vi "Dir Buttons.vi"(1 "Direction 2":T2) -> (0 "Buttons Control":T1)   [LabVIEW 2015]
uses:
  DIR GAME.ctl
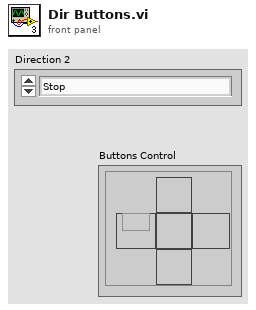
[diagram p1: front panel]
types:
  T1 = cluster{"Front":bool, "Right":bool, "Back":bool, "Left":bool, "Stop":bool}
  T2 = typedef "DIR GAME.ctl" = enum16{"Stop", "Front", "FR", "Right", "BR", "Back", "BL", "Left", "FL"}
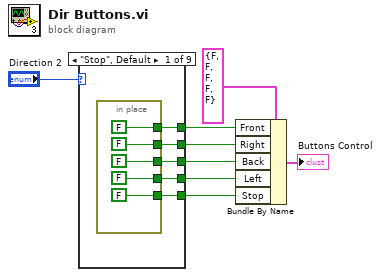
[diagram p0: block diagram]
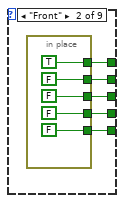
[diagram p2: hidden frame]
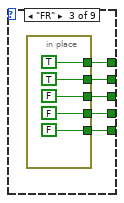
[diagram p3: hidden frame]
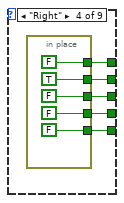
[diagram p4: hidden frame]
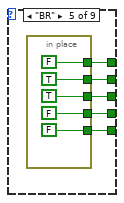
[diagram p5: hidden frame]
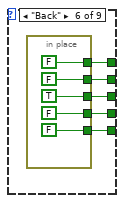
[diagram p6: hidden frame]
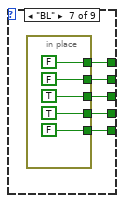
[diagram p7: hidden frame]
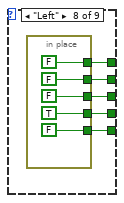
[diagram p8: hidden frame]
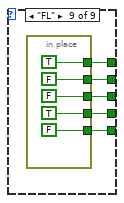
[diagram p9: hidden frame]
diagram:
  n1 = case shown="\"Stop\", Default" "Direction 2" {
    tunnel: [w13 w23 w33 w43 w53 w63 w73 w83 w93] -> w5
    tunnel: [w12 w22 w32 w42 w52 w62 w72 w82 w92] -> w4
    tunnel: [w11 w21 w31 w41 w51 w61 w71 w81 w91] -> w3
    tunnel: [w10 w20 w30 w40 w50 w60 w70 w80 w90] -> w2
    tunnel: [w9 w19 w29 w39 w49 w59 w69 w79 w89] -> w1
    frame "Stop", Default {
      n2 = in-place {
        in-place-border: [FALSE ("Front")] -> w13
        in-place-border: [FALSE ("Right")] -> w12
        in-place-border: [FALSE ("Back")] -> w11
        in-place-border: [FALSE ("Left")] -> w10
        in-place-border: [FALSE ("Stop")] -> w9
      }
    }
    frame "Front" {
      n3 = in-place {
        in-place-border: [TRUE ("Front")] -> w23
        in-place-border: [FALSE ("Right")] -> w22
        in-place-border: [FALSE ("Back")] -> w21
        in-place-border: [FALSE ("Left")] -> w20
        in-place-border: [FALSE ("Stop")] -> w19
      }
    }
    frame "FR" {
      n4 = in-place {
        in-place-border: [TRUE ("Front")] -> w33
        in-place-border: [TRUE ("Right")] -> w32
        in-place-border: [FALSE ("Back")] -> w31
        in-place-border: [FALSE ("Left")] -> w30
        in-place-border: [FALSE ("Stop")] -> w29
      }
    }
    frame "Right" {
      n5 = in-place {
        in-place-border: [FALSE ("Front")] -> w43
        in-place-border: [TRUE ("Right")] -> w42
        in-place-border: [FALSE ("Back")] -> w41
        in-place-border: [FALSE ("Left")] -> w40
        in-place-border: [FALSE ("Stop")] -> w39
      }
    }
    frame "BR" {
      n6 = in-place {
        in-place-border: [FALSE ("Front")] -> w53
        in-place-border: [TRUE ("Right")] -> w52
        in-place-border: [TRUE ("Back")] -> w51
        in-place-border: [FALSE ("Left")] -> w50
        in-place-border: [FALSE ("Stop")] -> w49
      }
    }
    frame "Back" {
      n7 = in-place {
        in-place-border: [FALSE ("Front")] -> w63
        in-place-border: [FALSE ("Right")] -> w62
        in-place-border: [TRUE ("Back")] -> w61
        in-place-border: [FALSE ("Left")] -> w60
        in-place-border: [FALSE ("Stop")] -> w59
      }
    }
    frame "BL" {
      n8 = in-place {
        in-place-border: [FALSE ("Front")] -> w73
        in-place-border: [FALSE ("Right")] -> w72
        in-place-border: [TRUE ("Back")] -> w71
        in-place-border: [TRUE ("Left")] -> w70
        in-place-border: [FALSE ("Stop")] -> w69
      }
    }
    frame "Left" {
      n9 = in-place {
        in-place-border: [FALSE ("Front")] -> w83
        in-place-border: [FALSE ("Right")] -> w82
        in-place-border: [FALSE ("Back")] -> w81
        in-place-border: [TRUE ("Left")] -> w80
        in-place-border: [FALSE ("Stop")] -> w79
      }
    }
    frame "FL" {
      n10 = in-place {
        in-place-border: [TRUE ("Front")] -> w93
        in-place-border: [FALSE ("Right")] -> w92
        in-place-border: [FALSE ("Back")] -> w91
        in-place-border: [TRUE ("Left")] -> w90
        in-place-border: [FALSE ("Stop")] -> w89
      }
    }
  }
  n11 = Bundle By Name(cluster=T1 {"Front"=FALSE, "Right"=FALSE, "Back"=FALSE, "Left"=FALSE, "Stop"=FALSE} ("Buttons Control 2"), "Front"=w5, "Right"=w4, "Back"=w3, "Left"=w2, "Stop"=w1) -> (→"Buttons Control":T1)
